vi "appendINIExtension.vi"(8 "error in (no error)":errorcluster {"code" format="Error %.0f"}, 11 "filepath":path caption="Configuration File Path") -> (0 "error out":errorcluster {"code" format="Error %.0f"}, 3 "filepathOut":path)   [LabVIEW 2017]
doc: "This VI appends the .ini file extension to an input filepath. If the .ini extension already exists, it returns the input path."
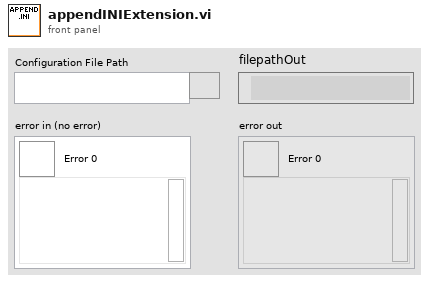
[diagram p1: front panel]
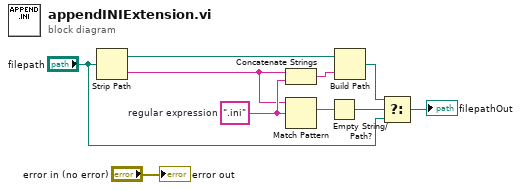
[diagram p0: block diagram]
diagram:
  w5 = ".ini"  # regular expression
  n1 = Strip Path(path="filepath") -> (stripped path=w7:path, name=w4:string)
  n2 = Concatenate Strings(w4, w5) -> (w6:string)
  n3 = Match Pattern(string=w4, regular expression=w5) -> (match substring=w9:string)  [unwired: 1 in, 3 out]
  n4 = Empty String/Path?(string/path=w9) -> (empty?=w8:bool)
  n5 = Build Path(base path=w7, name or relative path=w6) -> (appended path=w3:path)
  n6 = Select(t=w3, s=w8, f="filepath") -> (s? t:f=→"filepathOut":path)
  "error out" <- "error in (no error)"
